vi "Stop Clear.vi"(8 "error in (no error)":errorcluster, 11 "cetoni in":refnum<class "cetoni.lvclass">) -> (0 "error out":errorcluster, 3 "cetoni out":refnum<class "cetoni.lvclass">)   [LabVIEW 2018, in "cetoni.lvlib" / "cetoni.lvclass"]
uses:
  cetoni.lvclass
  Resources/GLOBAL/GLOBAL Time-critical.vi
  Program Files/cetoni/QmixSDK/lib/labview/labbCAN_Pump_API/labbCAN_Pump_API.lvlib
  <userlib>/QmixLib/QmixLib.lvlib
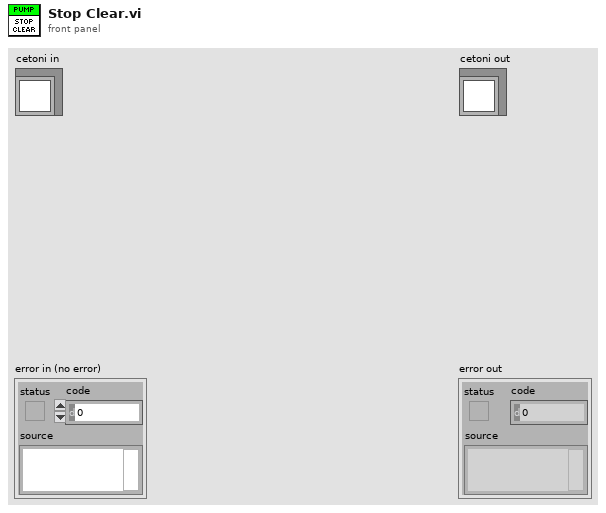
[diagram p1: front panel]
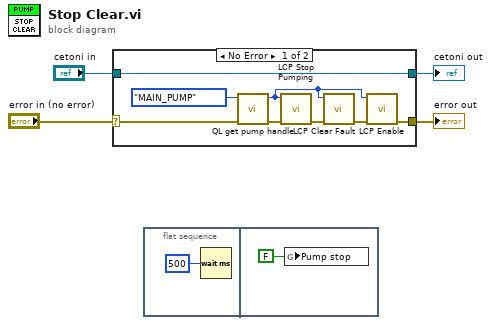
[diagram p0: block diagram]
diagram:
  n1 = case shown="No Error" "error in (no error)" {
    selector: "error in (no error)" -> [w8 w14]
    tunnel: [w9 w14] -> w3
    tunnel: [w12 w13] -> w1
    tunnel: "cetoni in" -> [w12 w13]
    frame No Error {
      n2 = call <userlib>:"QL get pump handle.vi"("error in (no error)"=w8, "pump"=enum16{"MAIN_PUMP"}."MAIN_PUMP") -> ("error out"=w7:errorcluster, "pump handle"=w6:u64)  [unwired: 8 in]
      n3 = call "LCP Stop Pumping.vi"("error in (no error)"=w7, "Pump Handle"=w6) -> ("error out"=w11:errorcluster)  [unwired: 9 in]
      n4 = call "LCP Clear Fault.vi"("error in (no error)"=w11, "Pump Handle"=w6) -> ("error out"=w10:errorcluster)  [unwired: 9 in]
      n5 = call "LCP Enable.vi"("error in (no error)"=w10, "Pump Handle"=w6) -> ("error out"=w9:errorcluster)  [unwired: 9 in]
    }
    frame Error {
    }
  }
  "error out" <- w3
  "cetoni out" <- w1
  n6 = flat-sequence {
    frame #0 {
      n7 = Wait (ms)(milliseconds to wait=u32 500) -> ()  [unwired: 1 out]
    }
    frame #1 {
      n8 = global write "GLOBAL Time-critical.vi" "Pump stop"(FALSE ("Pump stop")) -> ()
    }
  }
